vi "Send Email.vi"(0 "Sender's Name":string, 1 "Recipient's Name":string, 2 "Recipient's Email Address Address":string, 3 "Subject":string, 4 "Body":string) -> ()   [LabVIEW 2016]
panel:
  in  "CC Recipient (Optional)":string
  in  "Attachment - Optional":path
  in  "Port":i32=587
  in  "Enable SSL":bool=TRUE
  in  "Account Password":string="D4rtD0s3"
  in  "Account Username":string="dartmouth.epr.center"
  in  "Outgoing Mail Server (SMTP)":string="smtp.gmail.com"
  in  "Sender's Email Address":string="dartmouth.epr.center@gmail.com"
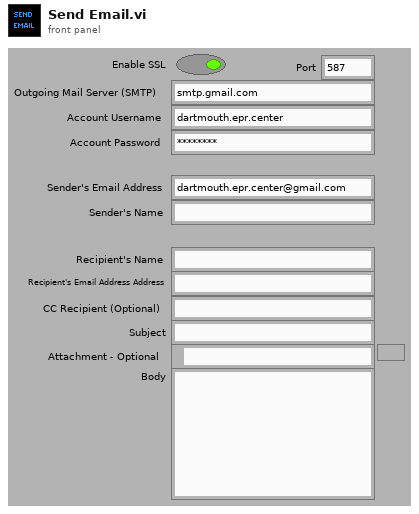
[diagram p1: front panel]
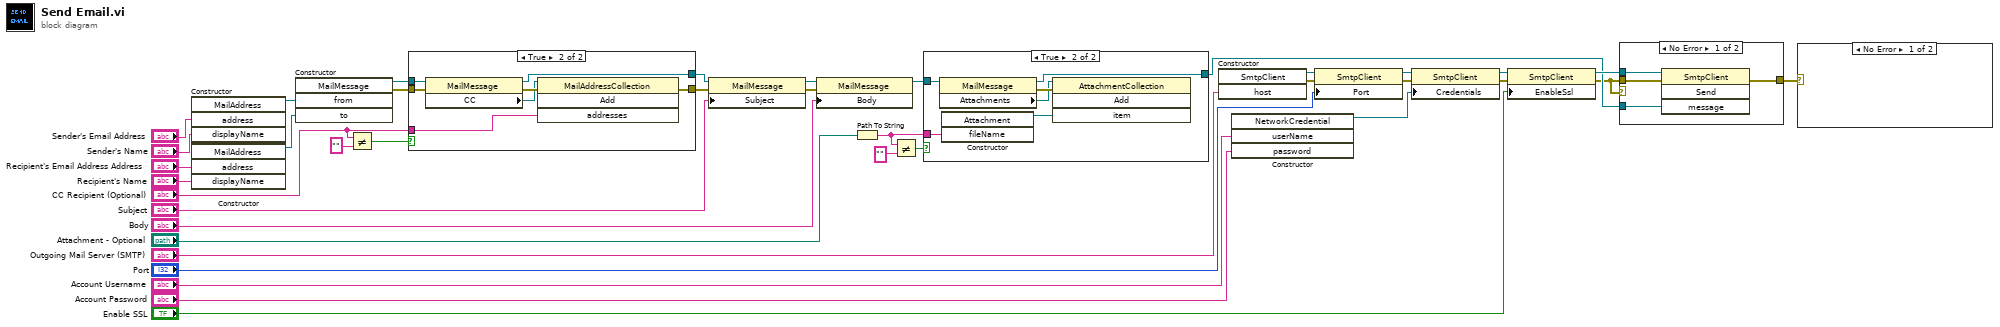
[diagram p0: block diagram]
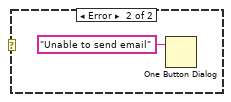
[diagram p2: hidden frame]
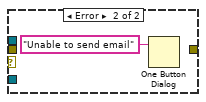
[diagram p3: hidden frame]
diagram:
  n1 = constructor class="MailAddress"("address"="Sender's Email Address", "displayName"="Sender's Name") -> (reference out=w37:refnum<k24>)  [unwired: 3 in, 4 out]
  n2 = constructor class="MailAddress"("address"="Recipient's Email Address Address", "displayName"="Recipient's Name") -> (reference out=w38:refnum<k24>)  [unwired: 3 in, 4 out]
  n3 = constructor class="MailMessage"("from"=w37, "to"=w38) -> (reference out=w7:refnum<k24>, error out=w6:errorcluster)  [unwired: 3 in, 3 out]
  n4 = Not Equal?(x="CC Recipient (Optional)", y="") -> (x != y?=w8:bool)
  n5 = case shown="True" w8 {
    tunnel: "CC Recipient (Optional)" -> [_ w45]
    tunnel: w7 -> [w40 w44]
    tunnel: w6 -> [w39 w43]
    tunnel: [w40 w42] -> w5
    tunnel: [w39 w41] -> w4
    frame False {
    }
    frame True {
      n6 = property class="MailMessage"(reference=w44, error in=w43) -> (reference out=w42:refnum<k24>, error out=w47:errorcluster, "CC"=w46:refnum<k24>)
      n7 = invoke class="MailAddressCollection" method="Add"(reference=w46, error in=w47, "addresses"=w45) -> (error out=w41:errorcluster)  [unwired: 1 in, 3 out]
    }
  }
  n8 = property class="MailMessage"(reference=w5, error in=w4, "Subject"="Subject") -> (reference out=w28:refnum<k24>, error out=w36:errorcluster)
  n9 = property class="MailMessage"(reference=w28, error in=w36, "Body"="Body") -> (reference out=w15:refnum<k24>)  [unwired: 1 out]
  n10 = Path To String(path="Attachment - Optional") -> (string=w10:string)
  n11 = Not Equal?(x=w10, y="") -> (x != y?=w11:bool)
  n12 = case shown="True" w11 {
    tunnel: w15 -> [w48 w51]
    tunnel: [w48 w50] -> w14
    tunnel: w10 -> [_ w49]
    frame False {
    }
    frame True {
      n13 = property class="MailMessage"(reference=w51) -> (reference out=w50:refnum<k24>, error out=w54:errorcluster, "Attachments"=w52:refnum<k24>)  [unwired: 1 in]
      n14 = constructor class="Attachment"("fileName"=w49) -> (reference out=w53:refnum<k24>)  [unwired: 3 in, 3 out]
      n15 = invoke class="AttachmentCollection" method="Add"(reference=w52, error in=w54, "item"=w53) -> ()  [unwired: 1 in, 4 out]
    }
  }
  n16 = constructor class="SmtpClient"("host"="Outgoing Mail Server (SMTP)") -> (reference out=w22:refnum<k24>, error out=w18:errorcluster)  [unwired: 3 in, 2 out]
  n17 = constructor class="NetworkCredential"("userName"="Account Username", "password"="Account Password") -> (reference out=w23:refnum<k24>)  [unwired: 3 in, 4 out]
  n18 = property class="SmtpClient"(reference=w22, error in=w18, "Port"="Port") -> (reference out=w21:refnum<k24>, error out=w17:errorcluster)
  n19 = property class="SmtpClient"(reference=w21, error in=w17, "Credentials"=w23) -> (reference out=w20:refnum<k24>, error out=w16:errorcluster)
  n20 = property class="SmtpClient"(reference=w20, error in=w16, "EnableSsl"="Enable SSL") -> (reference out=w19:refnum<k24>, error out=w2:errorcluster)
  n21 = case shown="No Error" w2 {
    tunnel: w19 -> [w58 _]
    tunnel: w2 -> [w57 _]
    tunnel: w14 -> [w56 _]
    tunnel: [w55 _] -> w1
    frame No Error {
      n22 = invoke class="SmtpClient" method="Send"(reference=w58, error in=w57, "message"=w56) -> (error out=w55:errorcluster)  [unwired: 1 in, 3 out]
    }
    frame Error {
      n23 = One Button Dialog(message="Unable to send email") -> ()  [unwired: 1 in, 1 out]
    }
  }
  n24 = case shown="No Error" w1 {
    frame No Error {
    }
    frame Error {
      n25 = One Button Dialog(message="Unable to send email") -> ()  [unwired: 1 in, 1 out]
    }
  }
